vi "Update Core.vi"(8 "error in (no error)":cluster{"状态":bool, "代码":i32, "源":string} caption="错误输入（无错误）", 11 "双风扇输入":refnum<class "Dual Fan.lvclass">) -> (0 "error out":cluster{"状态":bool, "代码":i32, "源":string} caption="错误输出", 3 "双风扇输出":refnum<class "Dual Fan.lvclass">)   [LabVIEW 2013, in "Dual Fan.lvlib" / "Dual Fan.lvclass"]
doc: "每次轮询间隔中，检查硬件故障并在必要时切换风扇。"
uses:
  Dual Fan.lvclass
  Fan Info.ctl
  Dual Fan.lvclass/Dual Fan.ctl
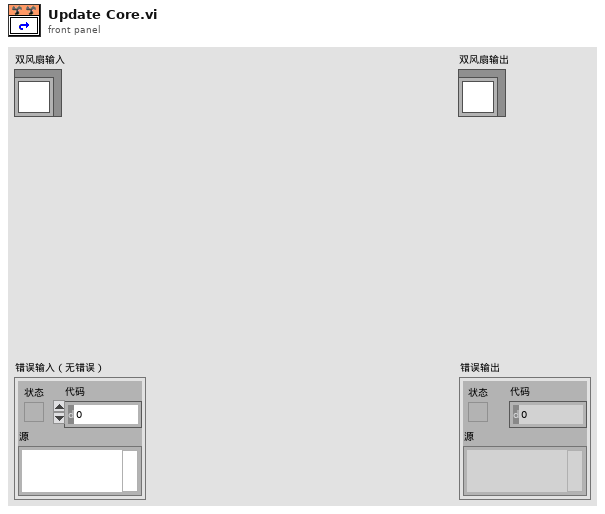
[diagram p1: front panel]
types:
  T1 = typedef "Dual Fan.lvlib/Dual Fan.lvclass/Fan Info.ctl" = cluster{"State":bool, "Fault":bool}
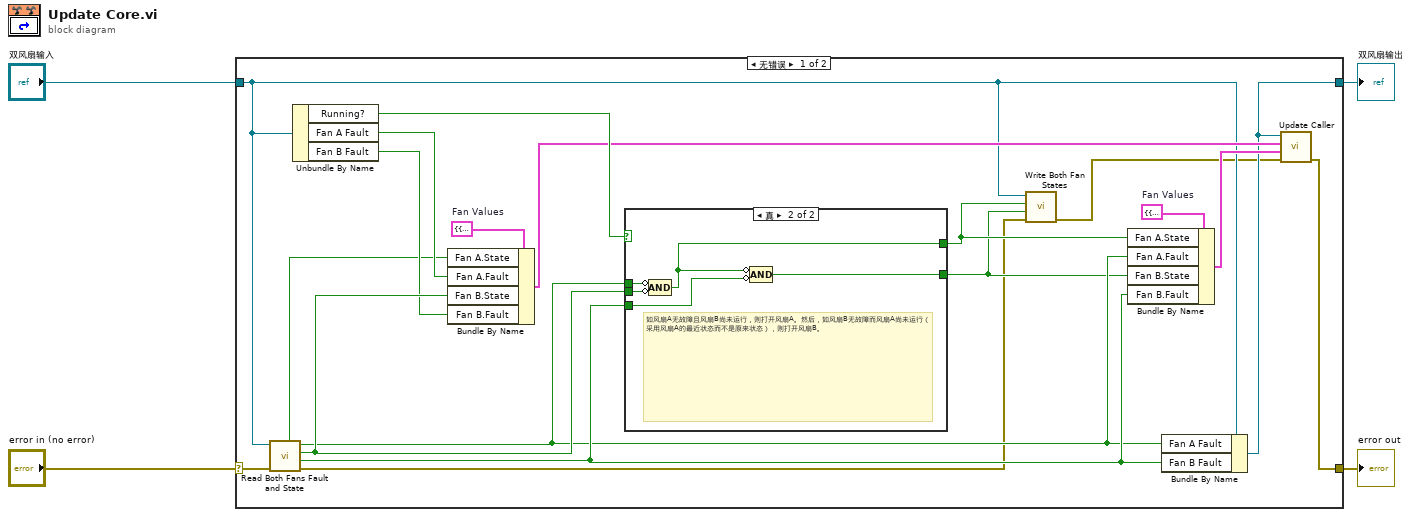
[diagram p0: block diagram]
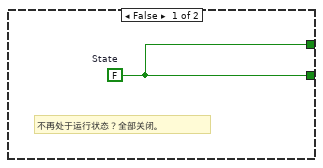
[diagram p2: hidden frame]
diagram:
  n1 = case shown="无错误" "error in (no error)" {
    selector: "error in (no error)" -> [w15 w31]
    tunnel: [w23 w31] -> w3
    tunnel: [w16 w30] -> w1
    tunnel: "双风扇输入" -> [w9 w30]
    frame No Error {
      w13 = cluster{"Fan A":T1, "Fan B":T1} {"Fan A"={"State"=FALSE, "Fault"=FALSE}, "Fan B"={"State"=FALSE, "Fault"=FALSE}}  # Fan Values
      w14 = cluster{"Fan A":T1, "Fan B":T1} {"Fan A"={"State"=FALSE, "Fault"=FALSE}, "Fan B"={"State"=FALSE, "Fault"=FALSE}}  # Fan Values
      n2 = call-dynamic "Read Both Fans Fault and State.vi"("error in (no error)"=w15, "双风扇输入"=w9) -> ("error out"=w5:cluster{"状态":bool, "代码":i32, "源":string}, "风扇B故障"=w11:bool, "风扇B状态"=w21:bool, "风扇A故障"=w10:bool, "风扇A状态"=w12:bool)  [unwired: 5 in]
      n3 = Unbundle By Name(w9) -> ("Running?"=w22:bool, "Fan A Fault"=w20:bool, "Fan B Fault"=w19:bool)
      n4 = Bundle By Name(cluster=w13, "Fan A.State"=w12, "Fan A.Fault"=w20, "Fan B.State"=w21, "Fan B.Fault"=w19) -> (w17:cluster{"Fan A":T1, "Fan B":T1})
      n5 = case shown="真" w22 {
        tunnel: w21 -> [_ w27]
        tunnel: w10 -> [_ w29]
        tunnel: w11 -> [_ w28]
        tunnel: [w24 w26] -> w8
        tunnel: [w24 w25] -> w7
        frame False {
          w24 = FALSE  # State
          # "不再处于运行状态？全部关闭。"
        }
        frame True {
          # "如风扇A无故障且风扇B尚未运行，则打开风扇A。然后，如风扇B无故障而风扇A尚未运行（采用风扇A的最近状态而不是原来状态），则打开风扇B。"
          n6 = Compound Arithmetic op=AND(invert w29, invert w27) -> (w26:bool)
          n7 = Compound Arithmetic op=AND(invert w26, invert w28) -> (w25:bool)
        }
      }
      n8 = call-dynamic "Write Both Fan States.vi"("error in (no error)"=w5, "风扇B状态"=w7, "风扇A状态"=w8, "双风扇输入"=w9) -> ("error out"=w6:cluster{"状态":bool, "代码":i32, "源":string})  [unwired: 7 in]
      n9 = Bundle By Name(cluster=w14, "Fan A.State"=w8, "Fan A.Fault"=w10, "Fan B.State"=w7, "Fan B.Fault"=w11) -> (w18:cluster{"Fan A":T1, "Fan B":T1})
      n10 = Bundle By Name(cluster=w9, "Fan A Fault"=w10, "Fan B Fault"=w11) -> (w16:refnum<class "Dual Fan.lvclass">)
      n11 = call "Update Caller.vi"("error in (no error)"=w6, "新值"=w18, "原值"=w17, "双风扇"=w16) -> ("error out"=w23:cluster{"状态":bool, "代码":i32, "源":string})  [unwired: 7 in]
    }
    frame Error {
    }
  }
  "error out" <- w3
  "双风扇输出" <- w1
